vi "Main.vi"() -> ()   [LabVIEW 2019]
doc: "The myRIO Project template acquires acceleration data from the onboard accelerometer and displays the changes of acceleration values in a waveform chart."
uses:
  <vilib>/myRIO/Common/Instrument Driver Framework/myRIO v1.0/Encoder/typedefs/Encoder Signal Mode.ctl
  <vilib>/myRIO/Instrument Drivers/Onboard IO/Encoder/typedefs/Encoder Reference.ctl
  <vilib>/myRIO/Common/Instrument Driver Framework/Utilities/typedefs/myRIO Generic Hardware Reference.ctl
  <vilib>/myRIO/Common/Instrument Driver Framework/Utilities/typedefs/Hardware Version Enum.ctl
  <vilib>/myRIO/Common/Instrument Driver Framework/Utilities/typedefs/myRIO v1.0 Reference.ctl
  <vilib>/myRIO/Common/Instrument Driver Framework/Utilities/typedefs/Generic FPGA Reference.ctl
  <vilib>/myRIO/Common/Instrument Driver Framework/myRIO v1.0/Encoder/typedefs/Encoder Channels Enum.ctl
  <vilib>/myRIO/Common/Instrument Driver Framework/myRIO v1.0/Encoder/typedefs/Encoder Configuration v1.0.ctl
  <vilib>/userDefined/High Color/nirio_resource_hc.ctl
  <vilib>/myRIO/Common/Instrument Driver Framework/Utilities/vis/Is FPGA Ref Available.vi
  <vilib>/myRIO/Common/Instrument Driver Framework/myRIO v1.0/Encoder/vis/myRIO v1.1 Open Encoder.vi
  <vilib>/myRIO/Instrument Drivers/Onboard IO/Encoder/vis/Read.vi
  <vilib>/myRIO/Common/Instrument Driver Framework/Utilities/vis/Validate Channels.vi
  <vilib>/myRIO/Common/Instrument Driver Framework/myRIO v1.0/Encoder/vis/myRIO v1.0 Reserve Encoder.vi
  <vilib>/myRIO/Common/Instrument Driver Framework/myRIO v1.0/UART/vis/myRIO v1.0 Close UART.vi
  <vilib>/myRIO/Common/Instrument Driver Framework/myRIO v1.0/Encoder/vis/myRIO v1.0 Build MUX Configuration Encoder.vi
  <vilib>/myRIO/Common/Instrument Driver Framework/myRIO v1.0/Resource Manager/vis/myRIO v1.0 Reserve Channel List.vi
  <vilib>/myRIO/Common/Instrument Driver Framework/myRIO v1.0/Resource Manager/vis/myRIO v1.0 Create Configuration List.vi
  <vilib>/myRIO/Common/Instrument Driver Framework/myRIO v1.0/Resource Manager/vis/myRIO v1.0 Reserve Channel.vi
  <vilib>/myRIO/Common/Instrument Driver Framework/myRIO v1.0/Resource Manager/vis/myRIO v1.0 Unreserve Channel.vi
  <vilib>/myRIO/Common/Instrument Driver Framework/myRIO v1.0/Resource Manager/vis/myRIO v1.0 Build Mutex Name.vi
  <vilib>/Utility/VariantDataType/GetNumericInfo.vi
  <vilib>/Utility/error.llb/Error Cluster From Error Code.vi
  <vilib>/myRIO/Common/Instrument Driver Framework/myRIO v1.0/myRIO v1.1 Open.vi
  <vilib>/myRIO/Common/Instrument Driver Framework/Utilities/vis/IO Manager.vi
  <vilib>/myRIO/Common/Instrument Driver Framework/Utilities/vis/Configuration Manager.vi
  <vilib>/myRIO/Common/Instrument Driver Framework/myRIO v1.0/Resource Manager/vis/myRIO v1.0 Configure IO.vi
  <vilib>/myRIO/Common/Instrument Driver Framework/myRIO v1.0/myRIO v1.0 Close.vi
  <vilib>/myRIO/Common/Instrument Driver Framework/myRIO v1.0/Encoder/vis/myRIO v1.0 Configure Encoder.vi
  <vilib>/myRIO/Common/Instrument Driver Framework/myRIO v1.0/Encoder/vis/myRIO v1.0 Read Encoder.vi
  <vilib>/Utility/file.llb/Write Delimited Spreadsheet (DBL).vi
  <vilib>/myRIO/Common/Instrument Driver Framework/Utilities/vis/FPGA Ref Manager.vi
  <vilib>/myRIO/Common/Instrument Driver Framework/myRIO v1.0/myRIO v1.0 Reset FPGA.vi
  <vilib>/myRIO/Common/Instrument Driver Framework/myRIO v1.0/IRQ/vis/myRIO v1.0 IRQ Info FGV.vi
  <vilib>/myRIO/Common/Instrument Driver Framework/myRIO v1.0/IRQ/vis/myRIO v1.0 Timer IRQ Info FGV.vi
  <vilib>/myRIO/Common/Instrument Driver Framework/myRIO v1.0/IRQ/vis/myRIO v1.0 ISR Agent.vi
  <vilib>/myRIO/Instrument Drivers/Utilities/vis/Reset Index.vi
  <vilib>/myRIO/Common/Instrument Driver Framework/myRIO v1.0/Resource Manager/vis/myRIO v1.0 Block Write Resource Manager.vi
  <vilib>/myRIO/Express VI/Onboard IO/Encoder/Encoder Express VI.xnode
  <vilib>/myRIO/Common/Instrument Driver Framework/myRIO v1.0/Encoder/typedefs/Encoder Count Direction Enum.ctl
  <vilib>/myRIO/Instrument Drivers/Onboard IO/Encoder/vis/myRIO Encoder Open.xnode
  <vilib>/myRIO/Instrument Drivers/Onboard IO/Encoder/Encoder.lvlib
  <vilib>/myRIO/Instrument Drivers/Utilities/Utilities.lvlib
panel:
  in  "Duty Cycle in 2":dbl=0.5
  out "error out":errorcluster
  in  "Stop":bool
  out "Direction":enum16{"Counting Up", "Counting Down"}(ring)
  out "Overflow?":bool
  in  "Reset":bool
  out "Graph":cluster{dbl, dbl}(graph)
  in  "Freq[Hz]":dbl=1000.0
  out "Direction 2":enum16{"Counting Up", "Counting Down"}(ring)
  out "Overflow? 2":bool
  in  "Reset 2":bool
  in  "K":dbl format="%#_13g"
  out "ref pos":dbl
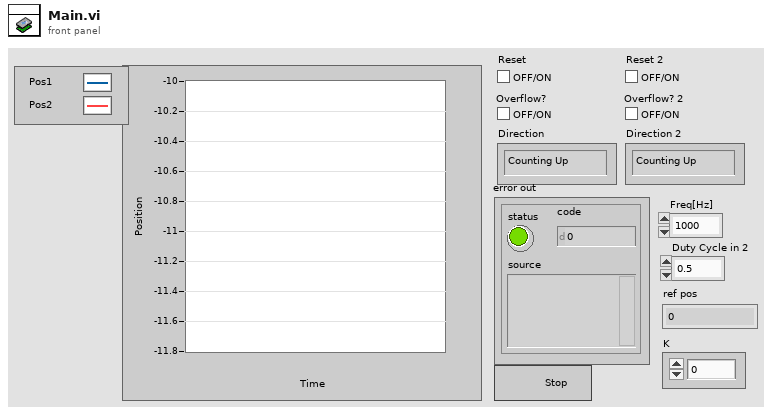
[diagram p1: front panel]
types:
  T1 = typedef "Encoder.lvlib/Encoder Reference.ctl" = cluster{"myRIO Reference":T2, "Encoder Channels Enum":T6}
  T2 = typedef "myRIO Generic Hardware Reference.ctl" = cluster{"myRIO Model":T3, "myRIO Hardware Reference":T4}
  T3 = typedef "Hardware Version Enum.ctl" = enum16{"Unknown", "myRIO-1900", "myRIO-1950", "roboRIO", "NI ELVIS RIO CM", "ELVIS III"}
  T4 = typedef "myRIO v1.0 Reference.ctl" = cluster{"Generic FPGA Reference":T5, "Allow multiple opens":bool}
  T5 = typedef "Generic FPGA Reference.ctl" = refnum<k20>
  T6 = typedef "Encoder Channels Enum.ctl" = enum16{"Not Connected", "C/ENC0", "C/ENC1", "A/ENC", "A/ENC0", "A/ENC1", "A/ENC2", "A/ENC3", "A/ENC4", "A/ENC5", "A/ENC6", "A/ENC7", "A/ENC8", "A/ENC9", "B/ENC", "B/ENC0", "B/ENC1", "B/ENC2", "B/ENC3", "B/ENC4", "B/ENC5", "B/ENC6", "B/ENC7", "B/ENC8", "B/ENC9", "DIO/ENC0", "DIO/ENC1", "DIO/ENC2", "DIO/ENC3", "DIO/ENC4"}
  T7 = typedef "Encoder Signal Mode.ctl" = enum16{"Quadrature phase signal", "Step and direction signal"}
  T8 = typedef "nirio_resource_hc.ctl" = tag
  T9 = typedef "Encoder Count Direction Enum.ctl" = enum16{"Counting Up", "Counting Down"}
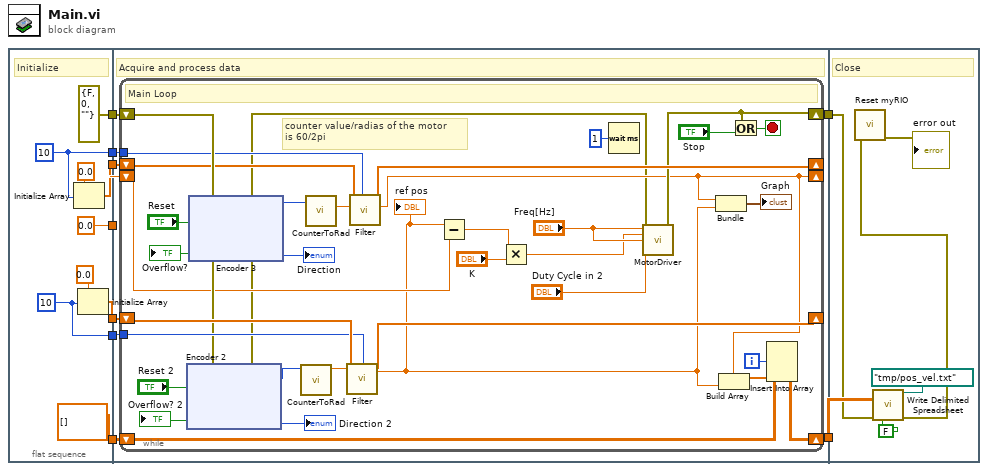
[diagram p0: block diagram]
diagram:
  n1 = flat-sequence {
    tunnel: [errorcluster {"status"=FALSE, "code"=0, "source"=""} ("error in (no error)")] -> w9
    tunnel: [0.0] -> w8
    tunnel: [dbl[][] [] ("array")] -> w7
    tunnel: [w14] -> w6
    tunnel: [w13] -> w5
    tunnel: [w11] -> w4
    tunnel: [w10] -> w3
    tunnel: w9 -> [w27]
    tunnel: w8 -> [w19]
    tunnel: w7 -> [w26]
    tunnel: [w25] -> w2
    tunnel: w6 -> [w24]
    tunnel: w5 -> [w23]
    tunnel: w4 -> [w22]
    tunnel: w3 -> [w21]
    tunnel: [w20] -> w1
    tunnel: w2 -> [w159]
    tunnel: w1 -> [w160]
    frame #0 {
      w10 = 10 ("dimension size")
      w14 = 10 ("dimension size")
      # "Initialize"
      n2 = Initialize Array(0.0 ("element"), w14) -> (w13:dbl[])
      n3 = Initialize Array(0.0 ("element"), w10) -> (w11:dbl[])
    }
    frame #1 {
      # "Acquire and process data"
      n4 = while {
        shift-right: [w40] -> w25
        shift-left: w27 -> [w53]
        shift-right: [w56] -> w20
        shift-left: w26 -> [w55]
        tunnel: w24 -> [w51]
        shift-right: [w49] -> _
        shift-left: w23 -> [w52]
        shift-right: [w45] -> _
        shift-left: w22 -> [w47]
        tunnel: w21 -> [w46]
        shift-right: [w35] -> _
        shift-left: w19 -> [w32]
        i -> [w50]
        stop <- w62 stop-if-true
        # "counter value/radias of the motor \nis 60/2pi"
        # "Main Loop"
        n5 = xnode "Encoder 3"("error in (no error)"=w53, "Reset Counter"="Reset") -> ("error out"=w36:errorcluster, "Counter Value"=w57:i32, "Counter Direction"=→"Direction":T9, "Overflow?"=→"Overflow?":bool)
        n6 = xnode "Encoder 2"("error in (no error)"=w36, "Reset Counter"="Reset 2") -> ("error out"=w28:errorcluster, "Counter Value"=w41:i32, "Counter Direction"=→"Direction 2":T9, "Overflow?"=→"Overflow? 2":bool)
        n7 = call "CounterToRad.vi"("Counter Value"=w41) -> ("rads"=w39:dbl)  [unwired: 10 in]
        n8 = call "CounterToRad.vi"("Counter Value"=w57) -> ("rads"=w48:dbl)  [unwired: 10 in]
        n9 = call "Filter.vi"("data"=w39, "Buffer Len"=w46, "Buffer in"=w47) -> ("ave out"=w31:dbl, "Buffer out"=w45:dbl[])  [unwired: 7 in]
        "ref pos" <- w31
        n10 = call "Filter.vi"("data"=w48, "Buffer Len"=w51, "Buffer in"=w52) -> ("ave out"=w35:dbl, "Buffer out"=w49:dbl[])  [unwired: 7 in]
        n11 = Subtract(x=w31, y=w32) -> (x-y=w33:dbl)
        n12 = Multiply(x=w33, y="K") -> (x*y=w30:dbl)
        n13 = Wait (ms)(milliseconds to wait=u32 1) -> ()  [unwired: 1 out]
        n14 = call "MotorDriver.vi"("Frequency [Hz]"="Freq[Hz]", "Duty Cycle in"=w30, "Frequency [Hz] 2"="Freq[Hz]", "Duty Cycle in 2"="Duty Cycle in 2", "error in (no error)"=w28) -> ("error out"=w40:errorcluster)  [unwired: 8 in, 2 out]
        n15 = Bundle("ave out"=w35, "ave out"=w31) -> (→"Graph":cluster{"ave out":dbl, "ave out":dbl})  [unwired: 1 in]
        n16 = Build Array(w35, w31) -> (w54:dbl[])
        n17 = Or(x=w40, y="Stop") -> (x .or. y?=w62:bool)
        n18 = Insert Into Array(array=w55, index (row)=w50, new element=w54) -> (w56:dbl[][])  [unwired: 1 in]
      }
    }
    frame #2 {
      # "Close"
      n19 = call-poly <vilib>:"Write Delimited Spreadsheet.vi"("file path (dialog if empty)"=path "/tmp/pos_vel.txt", "2D data"=w160, "error in (no error)"=w159, "transpose? (no:F)"=FALSE) -> ("error out"=w158:errorcluster)  [unwired: 10 in, 1 out]
      n20 = call <vilib>:"Reset myRIO.vi"("error in (no error)"=w158) -> ("error out"=→"error out":errorcluster)  [unwired: 10 in]
    }
  }
